vi "Write preparePass.vi"(8 "error in (no error)":errorcluster, 10 "preparePass":bool, 11 "PassTactic in":refnum<class "PassTactic.lvclass">) -> (0 "error out":errorcluster, 3 "PassTactic out":refnum<class "PassTactic.lvclass">)   [LabVIEW 2023, in "PassTactic.lvclass"]
uses:
  PassTactic.lvclass
  PassTactic.lvclass/PassTactic.ctl
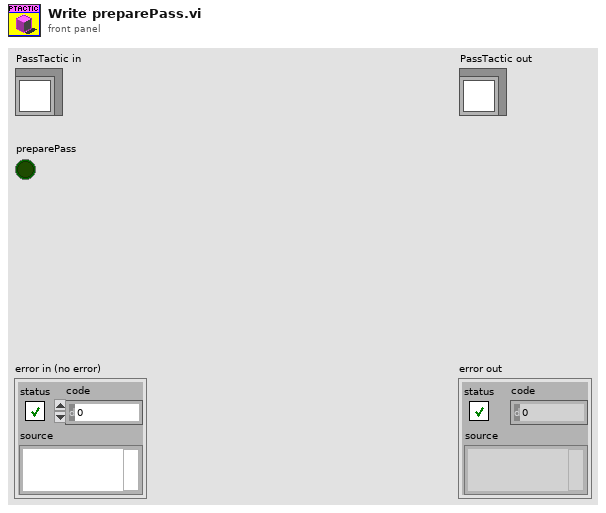
[diagram p1: front panel]
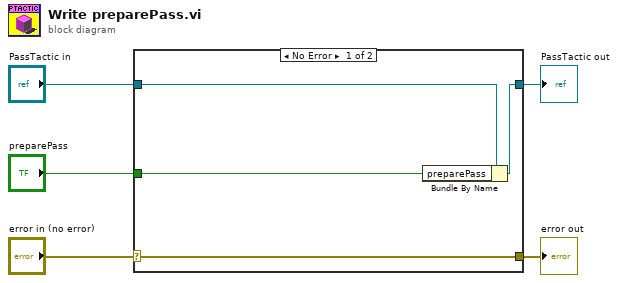
[diagram p0: block diagram]
diagram:
  n1 = case shown="No Error" "error in (no error)" {
    selector: "error in (no error)" -> [w9 w10]
    tunnel: [w9 w10] -> w4
    tunnel: [w7 w11] -> w2
    tunnel: "PassTactic in" -> [w8 w11]
    tunnel: "preparePass" -> [w6 _]
    frame No Error {
      n2 = Bundle By Name(cluster=w8, "preparePass"=w6) -> (w7:refnum<class "PassTactic.lvclass">)
    }
    frame Error {
    }
  }
  "error out" <- w4
  "PassTactic out" <- w2
